vi "MAIN_merFISH_photobleaching_injections.vi"(0 "Data cluster":T1, 1 "queue valve":refnum<queue>, 2 "queue pump":refnum<queue>, 7 "Valve H":u8(knob)=1 min=1 max=22 scale=1.0..22.0, 11 "error in":errorcluster, 12 "Photobleaching manager Refnum":refnum<vi>, 13 "Valve Refnum":refnum<vi>, 14 "Valve position OUT Refnum":refnum<vi>) -> (4 "Next task":T2, 15 "error out":errorcluster)   [LabVIEW 2015]
uses:
  CONTROLS/Q_main_element.ctl
  CONTROLS/Q_VALVE_element.ctl
  CONTROLS/Q_PUMP_element.ctl
  GLOBAL/Global_ABORT.vi
  GLOBAL/Global_VALVE.vi
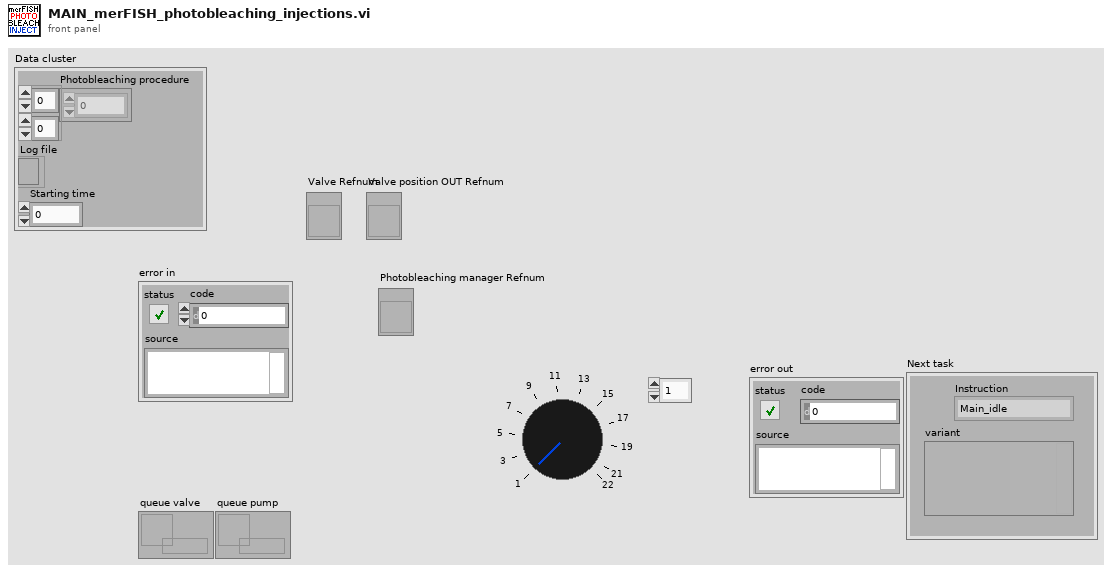
[diagram p1: front panel]
types:
  T1 = cluster{"Photobleaching procedure":i32[][], "Log file":refnum<file>, "Starting time":dbl}
  T2 = typedef "Q_main_element.ctl" = cluster{"variant":variant, "Instruction":enum16{"Main_idle", "Main_initialize", "Main_initialize_TDMS", "Main_initialize_Queue", "Main_error", "Main_DAQ_initialization_results", "Main_ASI_initialization_results", "Main_Piezo_initialization_results", "Main_Valve_initialization_results", "Main_Pump_initialization_results", "Main_CAMERA_initialization_results", "Main_FPGA_initialization_results", "Main_DAQ_error", "Main_ASI_error", "Main_Piezo_error", "Main_CAMERA_error", "Main_Valve_error", "Main_Pump_error", "Main_FPGA_error", "Main_start_acquiring", "Main_not_acquiring", "Main_acquiring", "Main_stop_acquiring", "Main_change_exposure", "Main_change_z_scan_parameters", "Main_define_ROI", "Main_define_mosaic", "Main_read_kinetic_time", "Main_cooler", "Main_read_temperature", "Main_save_XY", "Main_load_XY", "Main_discard_XY", "Main_move_to_XY", "Main_measure_QPD", "Main_autofocus_calibration", "Main_autofocus_initialization", "Main_autofocus_stop", "Main_save_PID", "Main_change_H_valve_position", "Main_two_way_valve", "Main_save_movie", "Main_init_single_scan", "Main_single_scan", "Main_stop_single_scan", "Main_merFISH_illumination_parameters", "Main_merFISH_buffer_probe_list", "Main_merFISH_injections_procedure", "Main_merFISH_save_setpoint", "Main_merFISH_DAPI_parameters", "Main_merFISH_Brightfield_parameters", "Main_merFISH_save_embryo_ROI", "Main_merFISH_init", "Main_merFISH_resume", "Main_merFISH_start_autofocus", "Main_merFISH_open_close_valve_merFISH", "Main_merFISH_open_close_valve_photobleaching", "Main_merFISH_hybridization", "Main_merFISH_move_to_ROI", "Main_merFISH_wait_stabilization", "Main_merFISH_move_to_REF", "Main_merFISH_scan", "Main_merFISH_photobleaching_injection", "Main_merFISH_photobleaching", "Main_merFISH_send_email", "Main_merFISH_close", "Main_STOP"}}
  T3 = cluster{"Pressure (mbar)":i32, "Volume (µl)":i32, "Flow rate (ul/s) ":i32}
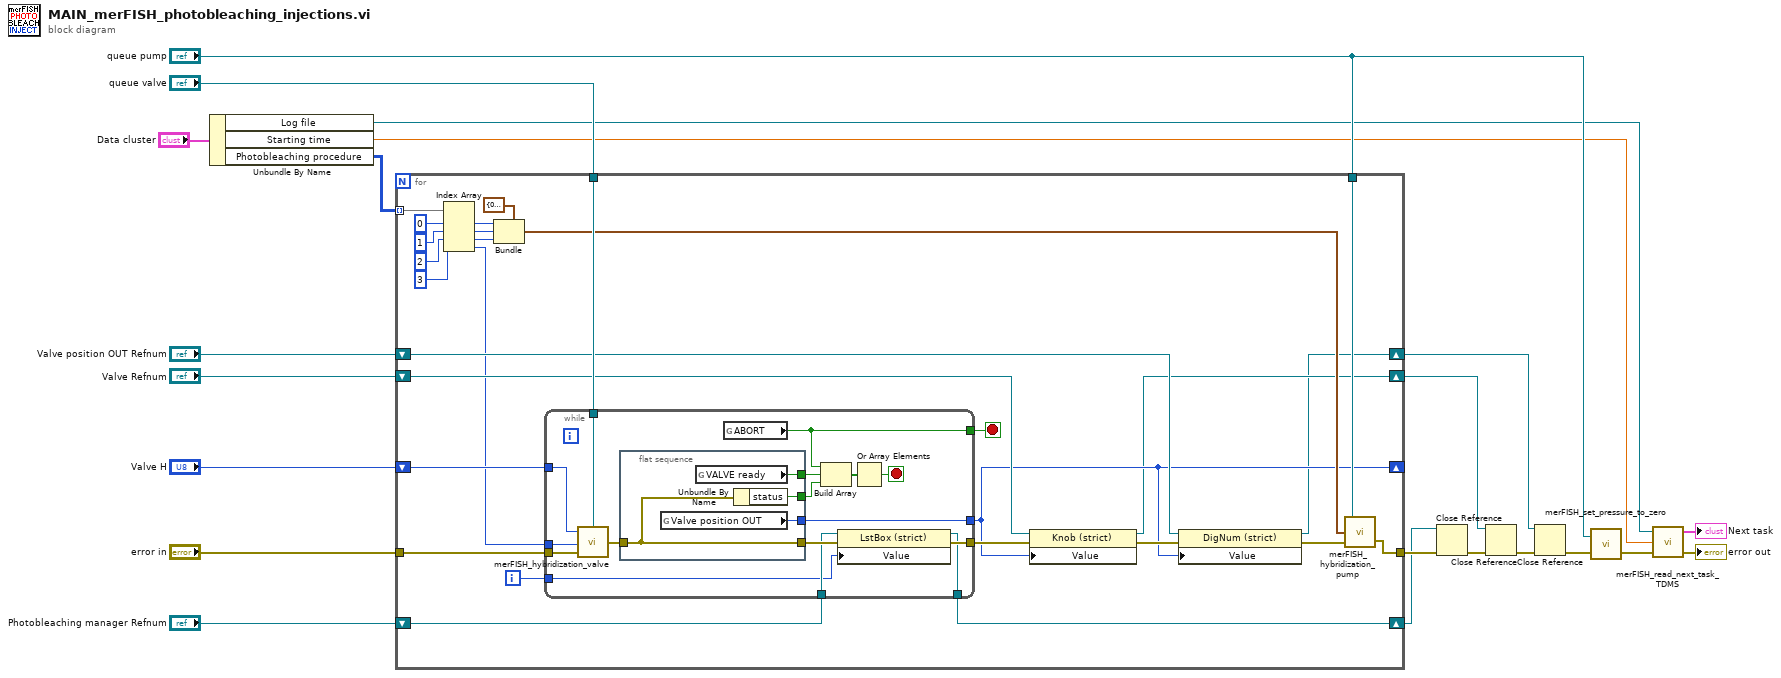
[diagram p0: block diagram]
diagram:
  n1 = Unbundle By Name("Data cluster") -> ("Log file"=w6:refnum<file>, "Starting time"=w5:dbl, "Photobleaching procedure"=w4:i32[][])
  n2 = for {
    tunnel: "queue valve" -> [w49]
    tunnel: "queue pump" -> [w42]
    tunnel: [w43] -> w12
    tunnel: w4 -> [w40] mode=indexing
    shift-right: [w27] -> _
    shift-left: "Valve H" -> [w38]
    tunnel: "error in" -> [w23]
    shift-right: [w32] -> w11
    shift-left: "Photobleaching manager Refnum" -> [w33]
    shift-right: [w25] -> w9
    shift-left: "Valve Refnum" -> [w30]
    shift-right: [w24] -> w7
    shift-left: "Valve position OUT Refnum" -> [w28]
    i -> [w37]
    stop <- w39 stop-if-true
    n3 = Index Array(array=w40, index #1=0 ("index"), index #2=1 ("index"), index #3=2 ("index"), index #4=3 ("index")) -> (element #1=w45:i32, element #2=w44:i32, element #3=w35:i32, element #4=w22:i32)
    n4 = Bundle(cluster=T3 {"Pressure (mbar)"=0, "Volume (µl)"=0, "Flow rate (ul/s) "=0} ("input data cluster"), "Pressure (mbar)"=w45, "Volume (µl)"=w44, "Flow rate (ul/s)"=w35) -> (w41:T3)
    n5 = while {
      tunnel: w49 -> [w65]
      tunnel: w23 -> [w64]
      tunnel: [w51] -> w31
      tunnel: w22 -> [w62]
      tunnel: [w57] -> w39
      tunnel: w38 -> [w61]
      tunnel: [w60] -> w27
      tunnel: w37 -> [w52]
      tunnel: w33 -> [w53]
      tunnel: [w50] -> w32
      stop <- w59 stop-if-true
      n6 = call "merFISH_hybridization_valve.vi"("queue valve"=w65, "error in"=w64, "New position"=w62, "Valve H"=w61) -> ("error out"=w63:errorcluster)
      n7 = flat-sequence {
        tunnel: w63 -> [w67]
        tunnel: [w67] -> w54
        tunnel: [w69] -> w60
        tunnel: [w68] -> w58
        tunnel: [w66] -> w55
        frame #0 {
          n8 = global read "Global_VALVE.vi" "Valve position OUT"() -> (w69:u8)
          n9 = global read "Global_VALVE.vi" "VALVE ready"() -> (w68:bool)
          n10 = Unbundle By Name(w67) -> ("status"=w66:bool)
        }
      }
      n11 = global read "Global_ABORT.vi" "ABORT"() -> (w57:bool)
      n12 = Build Array(w57, w58, w55) -> (w56:bool[])
      n13 = property class="LstBox (strict)"(reference=w53, error in=w54, "Value"=w52) -> (reference out=w50:refnum<vi>, error out=w51:errorcluster)
      n14 = Or Array Elements(Boolean array=w56) -> (logical OR=w59:bool)
    }
    n15 = property class="Knob (strict)"(reference=w30, error in=w31, "Value"=w27) -> (reference out=w25:refnum<vi>, error out=w29:errorcluster)
    n16 = property class="DigNum (strict)"(reference=w28, error in=w29, "Value"=w27) -> (reference out=w24:refnum<vi>, error out=w26:errorcluster)
    n17 = call "merFISH_hybridization_pump.vi"("error in"=w26, "input data cluster"=w41, "queue pump"=w42) -> ("error out"=w43:errorcluster)  [unwired: 1 in]
  }
  n18 = Close Reference(reference=w11, error in (no error)=w12) -> (error out=w10:errorcluster)
  n19 = Close Reference(reference=w9, error in (no error)=w10) -> (error out=w8:errorcluster)
  n20 = Close Reference(reference=w7, error in (no error)=w8) -> (error out=w2:errorcluster)
  n21 = call "merFISH_set_pressure_to_zero.vi"("error in"=w2, "queue pump"="queue pump") -> ("error out"=w21:errorcluster)  [unwired: 1 in]
  n22 = call "merFISH_read_next_task_TDMS.vi"("error in"=w21, "Starting time"=w5, "Log file"=w6) -> ("error out"=→"error out":errorcluster, "task"=→"Next task":T2)  [unwired: 1 in]
